vi "PPMS.Get Angle.vi"(8 "error in (no error)":errorcluster, 11 "instrument.PPMS":refnum<class "instrument.PPMS.lvclass">) -> (0 "error out":errorcluster, 2 "Angle (°)":dbl, 3 "instrument.PPMS out":refnum<class "instrument.PPMS.lvclass">)   [LabVIEW 2016, in "instrument.PPMS.lvclass"]
uses:
  instrument.PPMS.lvclass
  instrument.PPMS.lvclass/instrument.PPMS.ctl
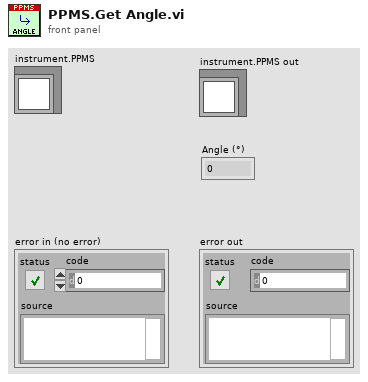
[diagram p1: front panel]
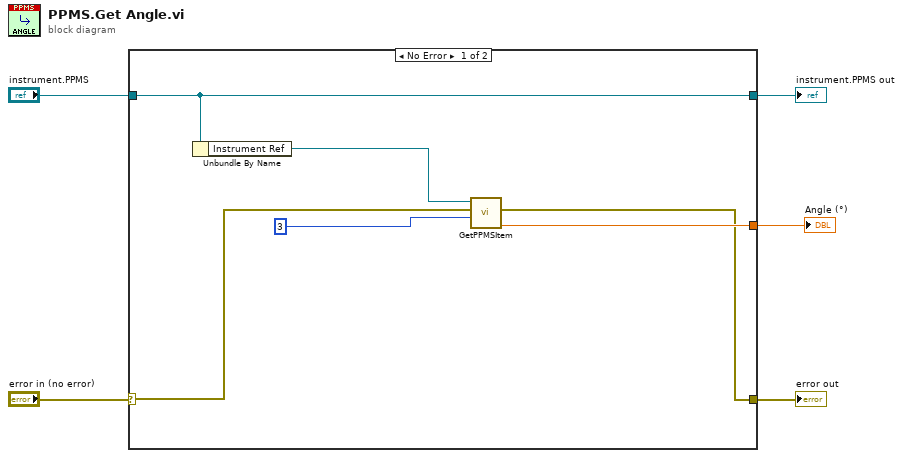
[diagram p0: block diagram]
diagram:
  n1 = case shown="No Error" "error in (no error)" {
    selector: "error in (no error)" -> [w8 w13]
    tunnel: [w7 w13] -> w5
    tunnel: "instrument.PPMS" -> [w11 w12]
    tunnel: [w11 w12] -> w2
    tunnel: [w9 _] -> w1
    frame No Error {
      n2 = Unbundle By Name(w11) -> ("Instrument Ref"=w6:refnum<k24>)
      n3 = call "GetPPMSItem.vi"("Channel"=3, "error in (no error)"=w8, "Instrument Ref In"=w6) -> ("Result"=w9:dbl, "error out"=w7:errorcluster)  [unwired: 1 in, 2 out]
    }
    frame Error {
    }
  }
  "Angle (°)" <- w1
  "error out" <- w5
  "instrument.PPMS out" <- w2
